vi "OnLoadNextGame.vi"(8 "error in (no error)":errorcluster, 11 "Menu in":refnum<class "Menu.lvclass">) -> (0 "error out":errorcluster, 3 "Menu out":refnum<class "Menu.lvclass">)   [LabVIEW 2019, in "RT_Game.lvlib" / "Menu.lvclass"]
uses:
  Menu.lvclass
  Game/Game.lvclass
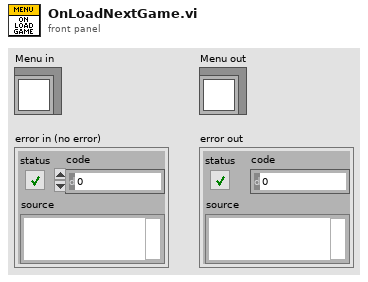
[diagram p1: front panel]
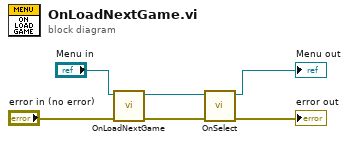
[diagram p0: block diagram]
diagram:
  n1 = call-parent "OnLoadNextGame.vi"("error in (no error)"="error in (no error)", "Game in"="Menu in") -> ("error out"=w6:errorcluster, "Game out"=w2:refnum<class "Menu.lvclass">)  [unwired: 8 in]
  n2 = call-dynamic "OnSelect.vi"("error in (no error)"=w6, "Menu in"=w2) -> ("error out"=→"error out":errorcluster, "Menu out"=→"Menu out":refnum<class "Menu.lvclass">)  [unwired: 8 in]
